vi "TestExec.File Sync Config.vi"(9 "Dialog":bool, 11 "Config Folder":path=path "C:/MTE/Test Executive/Config") -> (1 "Changed":bool)   [LabVIEW 2018]
uses:
  TestExec.File Sync Config Data.ctl
  <vilib>/KATE/Queues/Queue Utils.lvlib
  <vilib>/KATE/Files/File Utils.lvlib
panel:
  out "Tab Control":enum32{"Inputs", "Data", "Outputs"}(tab)=enum."Data"
  out "CfgFileExists":bool
  in  "Sync Now":bool
  in  "Sync Enabled":bool
  in  "Sync Items":T1(array[cluster])
  in  "Save":bool
  in  "Cancel":bool
  out "Sync Config File":path
  in  "Reload":bool
  out "Sync Config":T2
  # "File Sync Config"
  # "Path Types:\nSource    \tDestination     \tOutcome\nFILE          \tFILE\t\t                  The source file will be copied to the destination file.\nFILE\t     \t    FOLDER\t\t          The source file will be copied into the destination folder.\nFOLDER\t   FOLDER\t\t          All files and subfolders of the source folder will be copied into the destination folder. \nFOLDER\t   FILE\t            \t     This is an invalid combination.  An error will be generated."
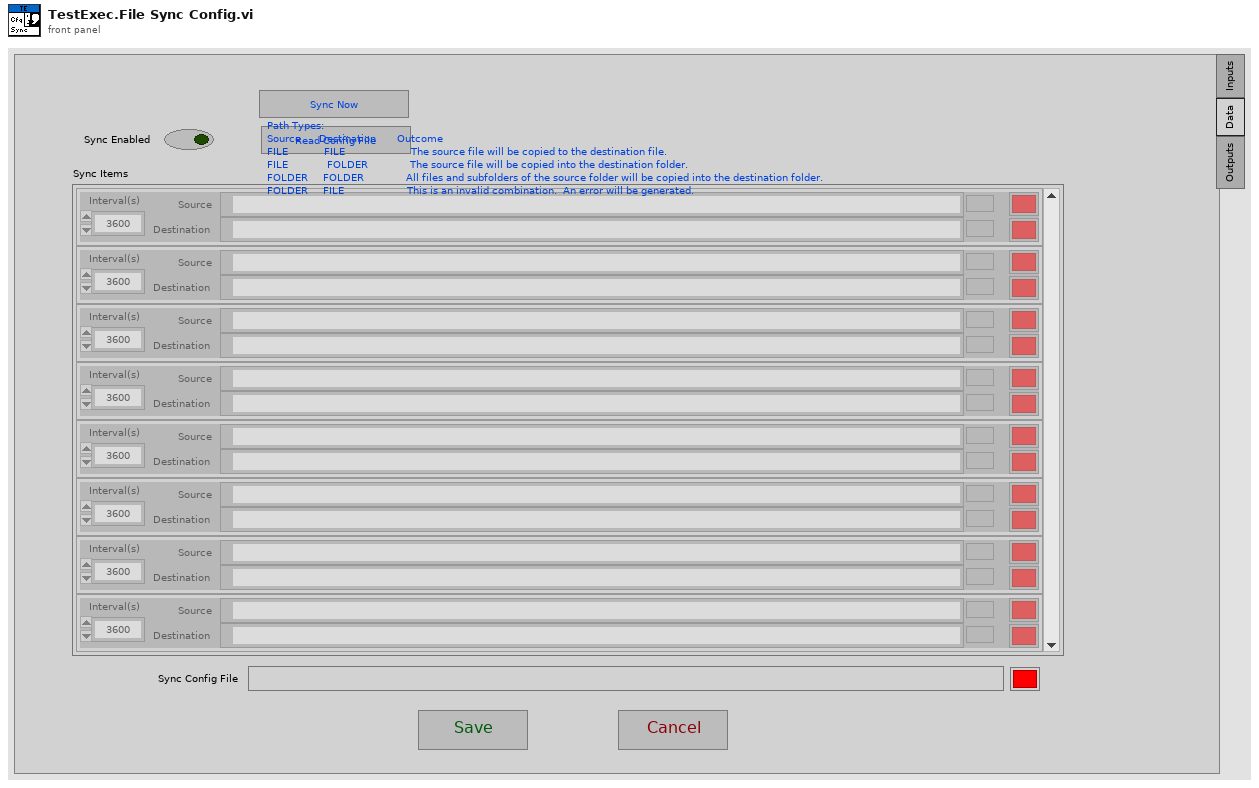
[diagram p1: front panel]
types:
  T1 = cluster{"Interval(s)":dbl, "Source":path, "Destination":path, "DestExists":bool, "SourceExists":bool}[]
  T2 = typedef "TestExec.File Sync Config Data.ctl" = cluster{"SyncEnabled":bool, "SyncItems":cluster{"Interval(s)":dbl, "Source":path, "Destination":path}[]}
  T3 = enum32{"Invalid", "Standard", "Closed", "Hidden", "Minimized", "Maximized"}
  T4 = cluster{"Enable":bool, "Files":cluster{"Interval":dbl, "Source":string, "Destination":string}[]}
  T5 = cluster{"Interval":dbl, "Source":string, "Destination":string}
  T6 = cluster{"Interval(s)":dbl, "Source":path, "Destination":path}
  T7 = cluster{"Interval(s)":dbl, "Source":path, "Destination":path, "DestExists":bool, "SourceExists":bool}
  T8 = cluster{"Config Folder":path, "Config File":path, "Sync Config":T2, "Canceled":bool}
  T9 = cluster{"Interval":dbl, "Source":string, "Destination":string}[]
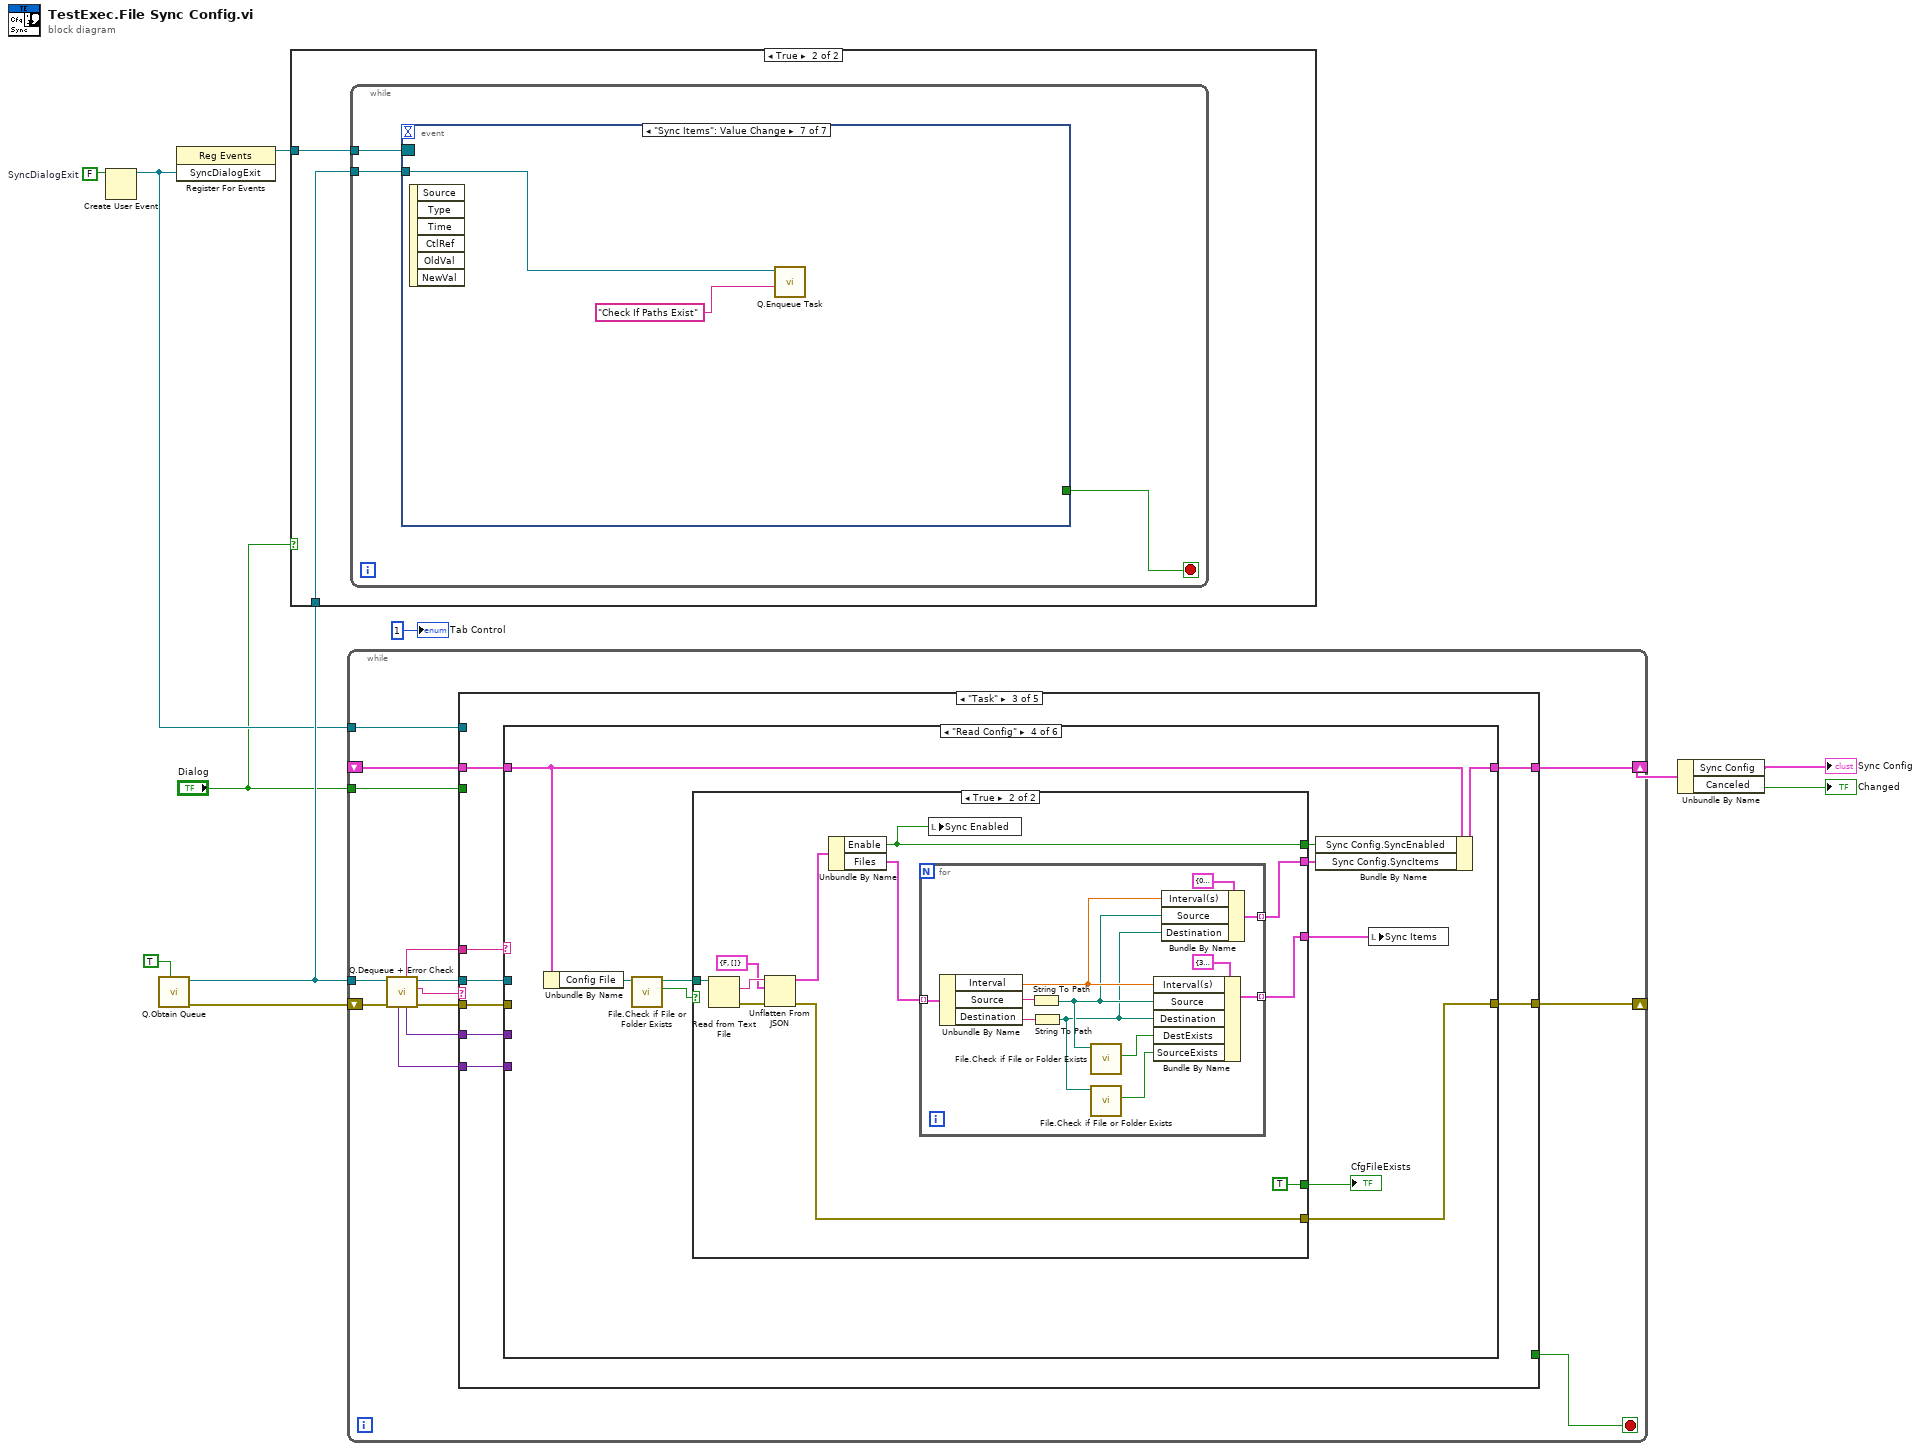
[diagram p0: block diagram]
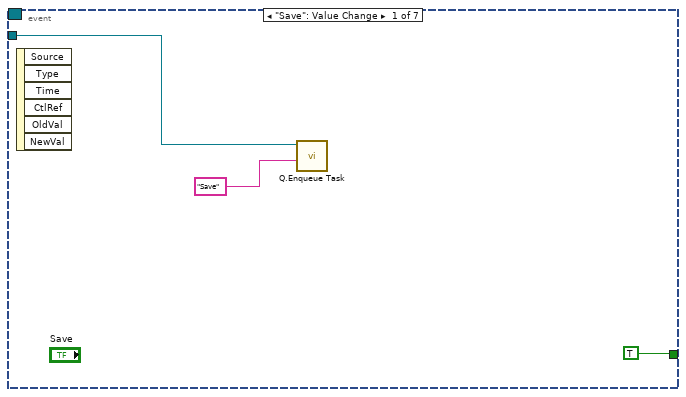
[diagram p3: hidden frame]
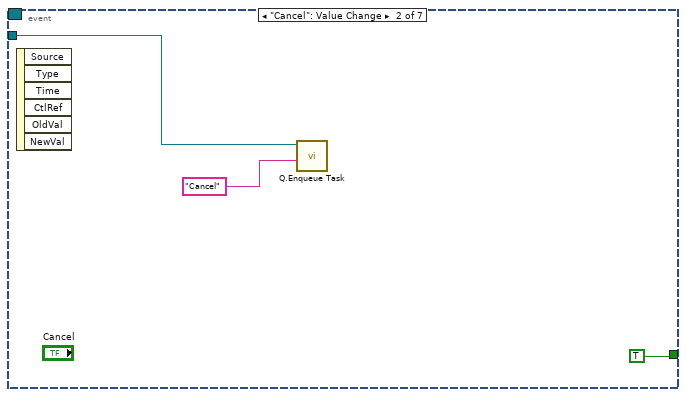
[diagram p4: hidden frame]
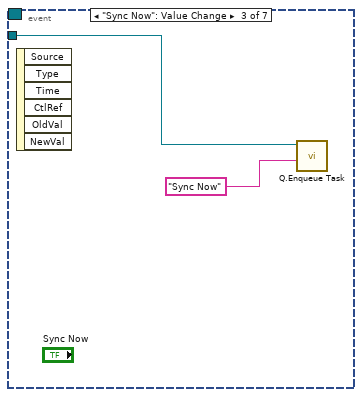
[diagram p5: hidden frame]
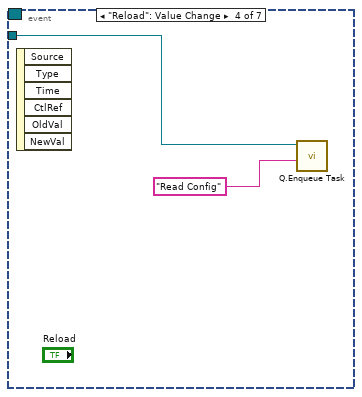
[diagram p6: hidden frame]
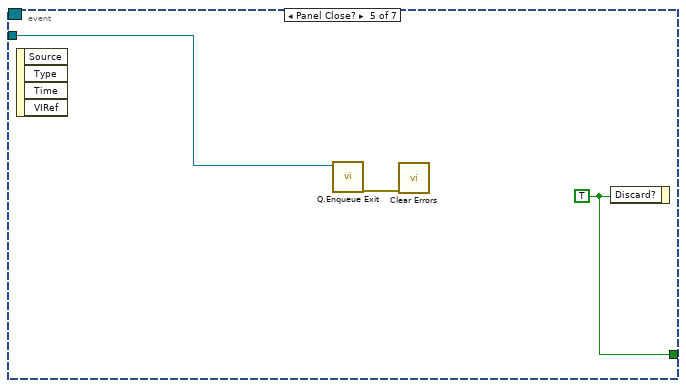
[diagram p7: hidden frame]
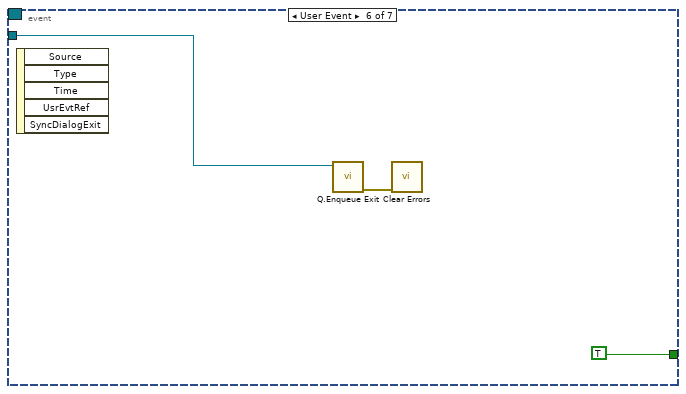
[diagram p8: hidden frame]
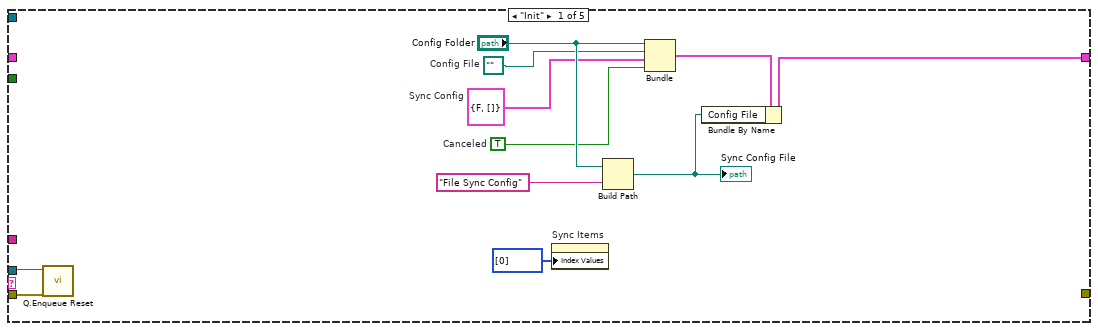
[diagram p9: hidden frame]
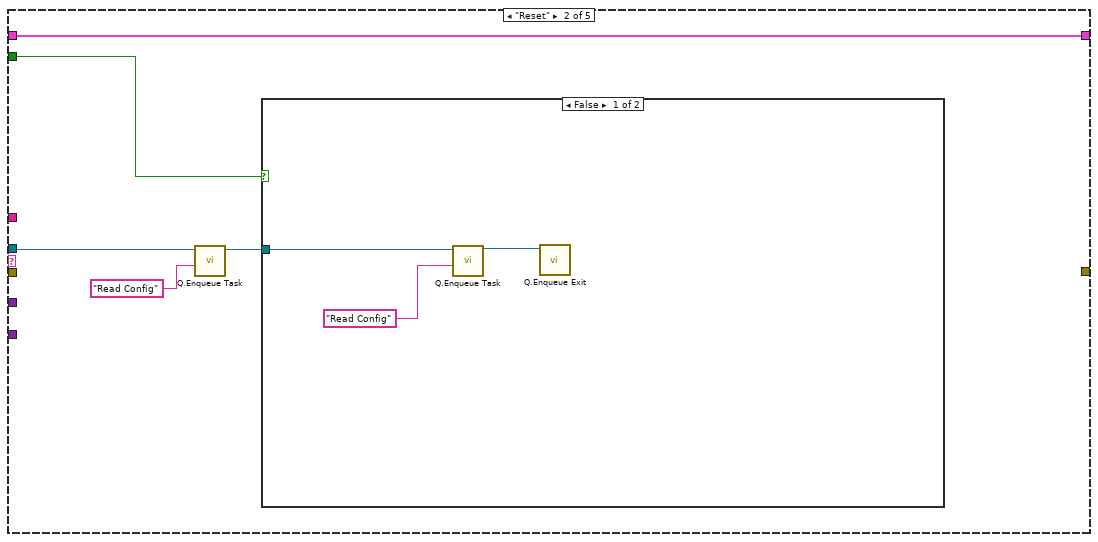
[diagram p10: hidden frame]
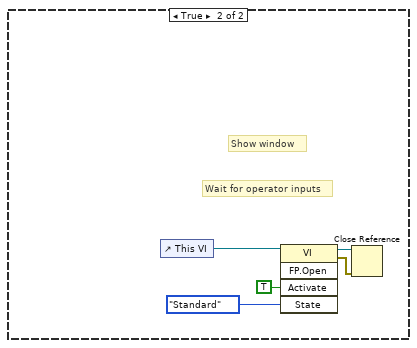
[diagram p11: hidden frame]
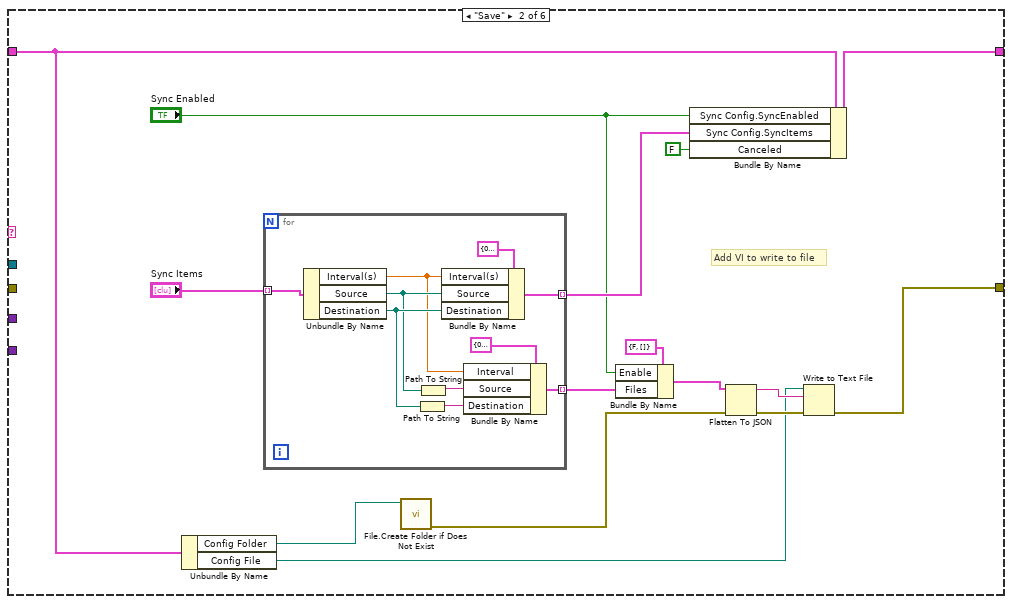
[diagram p13: hidden frame]
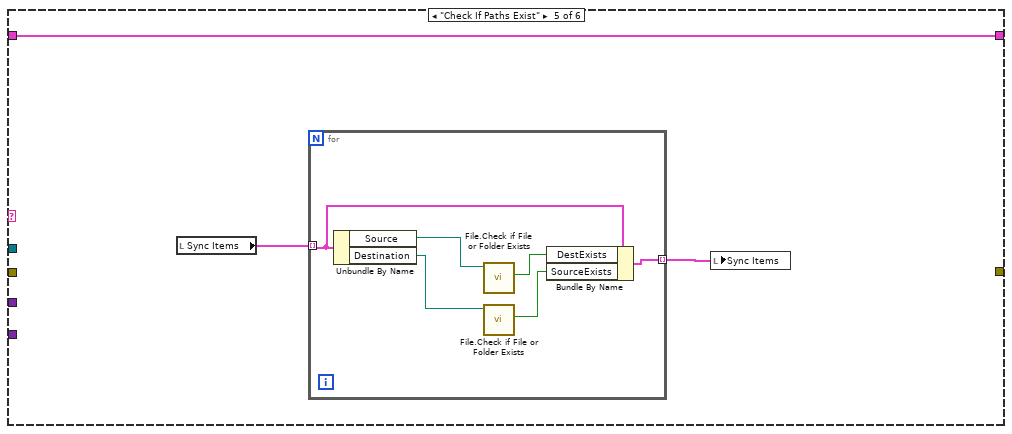
[diagram p16: hidden frame]
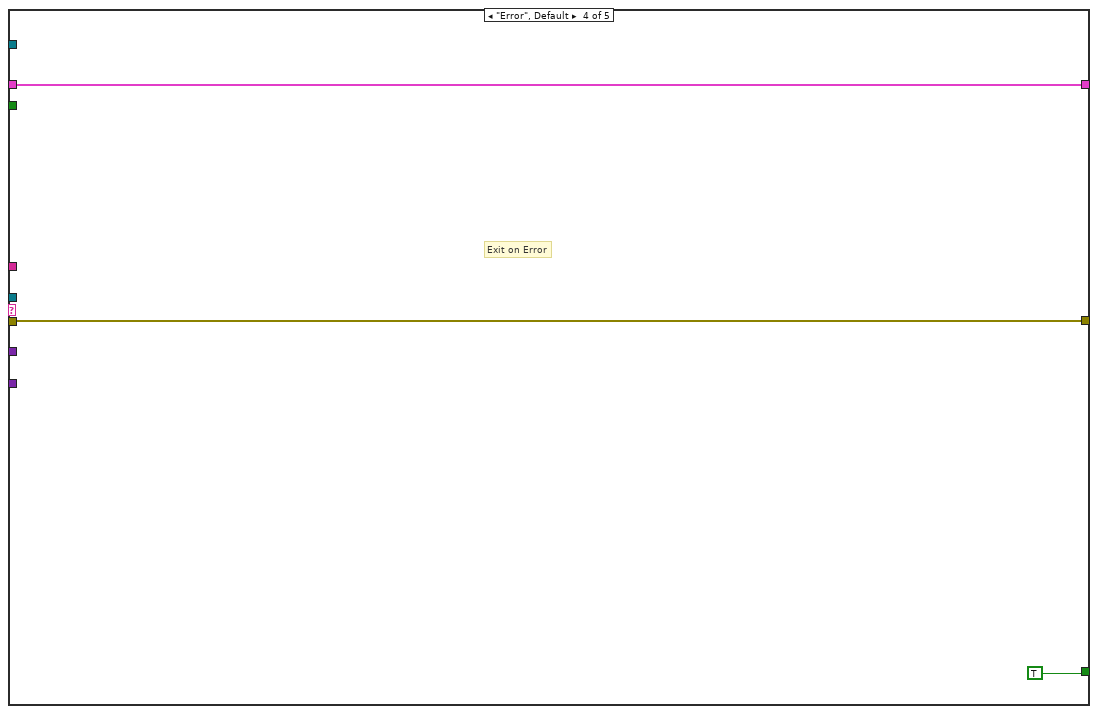
[diagram p18: hidden frame]
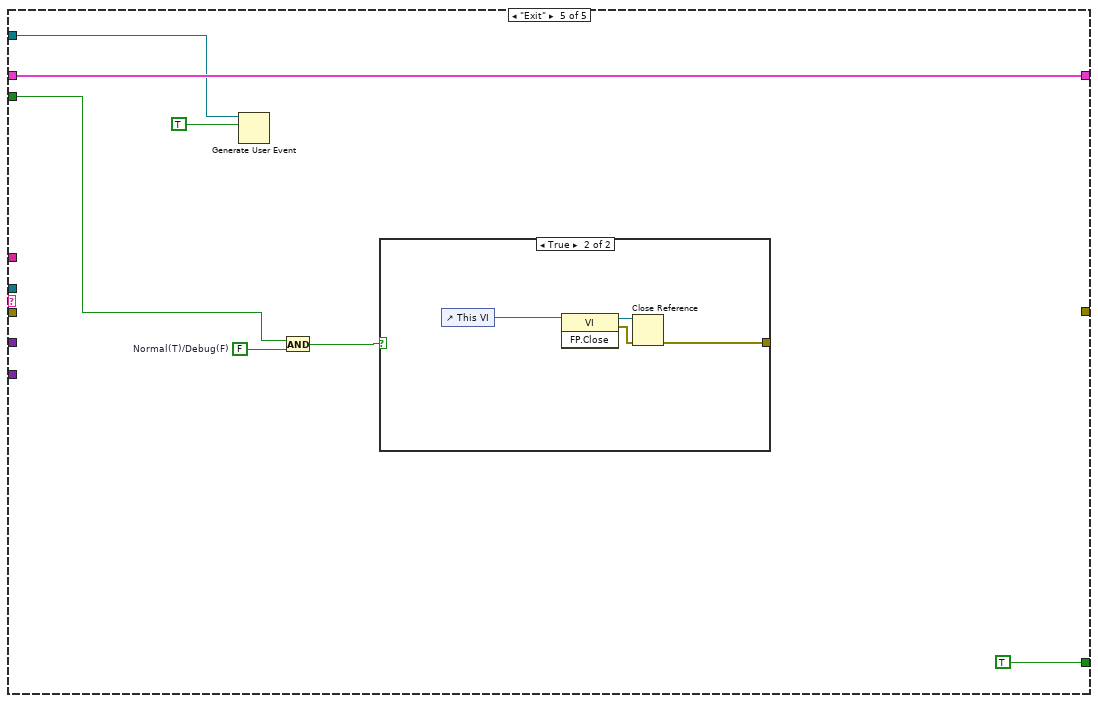
[diagram p19: hidden frame]
diagram:
  w11 = FALSE  # SyncDialogExit
  n1 = Create User Event(user event datatype=w11) -> (user event=w5:refnum<user-event>)  [unwired: 1 in, 1 out]
  n2 = call <vilib>:"Q.Obtain Queue.vi"("Enqueue Init"=TRUE) -> ("error out"=w7:errorcluster, "Q Out"=w6:refnum<queue>)  [unwired: 8 in, 1 out]
  n3 = register-events(w5) -> (reference out=w10:refnum<event-registration>)  [unwired: 2 in, 1 out]
  n4 = case shown="True" "Dialog" {
    tunnel: w10 -> [_ w13]
    tunnel: w6 -> [_ w12]
    frame False {
    }
    frame True {
      n5 = while {
        tunnel: w13 -> [w16]
        tunnel: w12 -> [w15]
        stop <- w14 stop-if-true
        n6 = event shown="[6] \"Sync Items\": Value Change" {
          selector: w16 -> [_ _ _ _ _ _ _]
          dyn-events: _ -> [_ _ _ _ _ _ _]
          timeout: _ -> [_ _ _ _ _ _ _]
          tunnel: w15 -> [w18 w21 w23 w25 w28 w31 w33]
          tunnel: [TRUE TRUE _ _ w29 TRUE _] -> w14
          event "Save": Value Change {
            n7 = event-data() -> ()  [unwired: 1 in, 6 out]
            n8 = call <vilib>:"Q.Enqueue Task.vi"("Task Name"="Save", "Q In"=w18) -> ()  [unwired: 8 in, 2 out]
          }
          event "Cancel": Value Change {
            n9 = event-data() -> ()  [unwired: 1 in, 6 out]
            n10 = call <vilib>:"Q.Enqueue Task.vi"("Task Name"="Cancel", "Q In"=w21) -> ()  [unwired: 8 in, 2 out]
          }
          event "Sync Now": Value Change {
            n11 = event-data() -> ()  [unwired: 1 in, 6 out]
            n12 = call <vilib>:"Q.Enqueue Task.vi"("Task Name"="Sync Now", "Q In"=w23) -> ()  [unwired: 8 in, 2 out]
          }
          event "Reload": Value Change {
            n13 = event-data() -> ()  [unwired: 1 in, 6 out]
            n14 = call <vilib>:"Q.Enqueue Task.vi"("Task Name"="Read Config", "Q In"=w25) -> ()  [unwired: 8 in, 2 out]
          }
          event Panel Close? {
            w29 = TRUE
            n15 = event-data() -> ()  [unwired: 1 in, 4 out]
            n16 = call <vilib>:"Q.Enqueue Exit.vi"("Q In"=w28) -> ("error out"=w27:errorcluster)  [unwired: 9 in, 1 out]
            n17 = call <vilib>:"Clear Errors.vi"("error in (no error)"=w27) -> ()  [unwired: 5 in, 2 out]
            n18 = event-data("Discard?"=w29) -> ()  [unwired: 1 in, 1 out]
          }
          event User Event {
            n19 = event-data() -> ()  [unwired: 1 in, 5 out]
            n20 = call <vilib>:"Q.Enqueue Exit.vi"("Q In"=w31) -> ("error out"=w30:errorcluster)  [unwired: 9 in, 1 out]
            n21 = call <vilib>:"Clear Errors.vi"("error in (no error)"=w30) -> ()  [unwired: 5 in, 2 out]
          }
          event "Sync Items": Value Change {
            n22 = event-data() -> ()  [unwired: 1 in, 6 out]
            n23 = call <vilib>:"Q.Enqueue Task.vi"("Task Name"="Check If Paths Exist", "Q In"=w33) -> ()  [unwired: 8 in, 2 out]
          }
        }
      }
    }
  }
  n24 = while {
    shift-right: [w40] -> _
    shift-left: w7 -> [w45]
    tunnel: w6 -> [w43]
    shift-right: [w38] -> w4
    shift-left: _ -> [w37]
    tunnel: w5 -> [w36]
    tunnel: "Dialog" -> [w35]
    stop <- w39 stop-if-true
    n25 = call <vilib>:"Q.Dequeue + Error Check.vi"("Error In"=w45, "Q In"=w43) -> ("error out"=w46:errorcluster, "Cmd"=w48:string, "Q Out"=w47:refnum<queue>, "Data1"=w42:variant, "Sub"=w44:string, "Data2"=w41:variant)  [unwired: 4 in]
    n26 = case shown="\"Task\"" w48 {
      tunnel: w47 -> [w49 w63 w79 _ _]
      tunnel: w46 -> [w50 _ w78 w152 _]
      tunnel: w44 -> [_ _ w80 _ _]
      tunnel: w42 -> [_ _ w77 _ _]
      tunnel: w41 -> [_ _ w76 _ _]
      tunnel: [_ _ w73 w152 _] -> w40
      tunnel: [_ _ _ TRUE TRUE] -> w39
      tunnel: [w58 w60 w74 w153 w159] -> w38
      tunnel: w37 -> [_ w60 w75 w153 w159]
      tunnel: w36 -> [_ _ _ _ w158]
      tunnel: w35 -> [_ w61 _ _ w154]
      frame "Init" {
        w52 = TRUE  # Canceled
        w55 = T2 {"SyncEnabled"=FALSE, "SyncItems"=[]}  # Sync Config
        w56 = path ""  # Config File
        n27 = call <vilib>:"Q.Enqueue Reset.vi"("Error In"=w50, "Q In"=w49) -> ()  [unwired: 8 in, 2 out]
        n28 = property on="Sync Items" class="Arr (strict)"("Index Values"=u32[] [0]) -> ()  [unwired: 2 in, 2 out]
        n29 = Build Path(base path="Config Folder", name or relative path="File Sync Config") -> (appended path=w54:path)
        "Sync Config File" <- w54
        n30 = Bundle("Config Folder"="Config Folder", "Config File"=w56, "Sync Config"=w55, "Canceled"=w52) -> (w59:T8)  [unwired: 1 in]
        n31 = Bundle By Name(cluster=w59, "Config File"=w54) -> (w58:T8)
      }
      frame "Reset" {
        n32 = call <vilib>:"Q.Enqueue Task.vi"("Task Name"="Read Config", "Q In"=w63) -> ("Q Out"=w62:refnum<queue>)  [unwired: 8 in, 1 out]
        n33 = case shown="False" w61 {
          tunnel: w62 -> [w66 _]
          frame False {
            n34 = call <vilib>:"Q.Enqueue Task.vi"("Task Name"="Read Config", "Q In"=w66) -> ("Q Out"=w65:refnum<queue>)  [unwired: 8 in, 1 out]
            n35 = call <vilib>:"Q.Enqueue Exit.vi"("Q In"=w65) -> ()  [unwired: 9 in, 2 out]
          }
          frame True {
            # "Show window"
            # "Wait for operator inputs"
            n36 = control-ref of="This VI"() -> (w72:refnum<vi>)
            n37 = invoke class="VI" method="FP.Open"(reference=w72, "Activate"=TRUE ("Activate?"), "State"=T3."Standard") -> (reference out=w71:refnum<vi>, error out=w70:errorcluster)  [unwired: 2 in, 3 out]
            n38 = Close Reference(reference=w71, error in (no error)=w70) -> ()  [unwired: 1 out]
          }
        }
      }
      frame "Task" {
        n39 = case shown="\"Read Config\"" w80 {
          tunnel: w79 -> [_ _ _ _ _ _]
          tunnel: w78 -> [_ _ _ _ _ _]
          tunnel: w77 -> [_ _ _ _ _ _]
          tunnel: w76 -> [_ _ _ _ _ _]
          tunnel: w75 -> [w81 w92 w107 w114 w143 w150]
          tunnel: [w81 w96 w107 w113 w143 w150] -> w74
          tunnel: [_ w86 _ w117 _ _] -> w73
          frame "Sync Now" {
            # "Add VI to perform Sync"
          }
          frame "Save" {
            # "Add VI to write to file"
            n40 = Unbundle By Name(w92) -> ("Config Folder"=w91:path, "Config File"=w87:path)
            n41 = for {
              tunnel: [w105] -> w93 mode=indexing
              tunnel: "Sync Items" -> [w104] mode=indexing
              tunnel: [w97] -> w84 mode=indexing
              n42 = Unbundle By Name(w104) -> ("Interval(s)"=w98:dbl, "Source"=w102:path, "Destination"=w103:path)
              n43 = Path To String(path=w103) -> (string=w100:string)
              n44 = Path To String(path=w102) -> (string=w101:string)
              n45 = Bundle By Name(cluster=T6 {"Interval(s)"=0.0, "Source"=path "", "Destination"=path ""} ("Sunc Config Item"), "Interval(s)"=w98, "Source"=w102, "Destination"=w103) -> (w105:T6)
              n46 = Bundle By Name(cluster=T5 {"Interval"=0.0, "Source"="", "Destination"=""} ("Sunc Config Item"), "Interval"=w98, "Source"=w101, "Destination"=w100) -> (w97:T5)
            }
            n47 = call <vilib>:"File.Create Folder if Does Not Exist.vi"("Path"=w91) -> ("error out"=w90:errorcluster)  [unwired: 8 in, 2 out]
            n48 = Bundle By Name(cluster=T4 {"Enable"=FALSE, "Files"=[]}, "Enable"="Sync Enabled", "Files"=w84) -> (w82:T4)
            n49 = Bundle By Name(cluster=w92, "Sync Config.SyncEnabled"="Sync Enabled", "Sync Config.SyncItems"=w93, "Canceled"=FALSE) -> (w96:T8)
            n50 = Flatten To JSON(anything=w82, error in (no error)=w90) -> (JSON string=w88:string, 11:w89:errorcluster)  [unwired: 1 in]
            n51 = Write to Text File(file (use dialog)=w87, text=w88, error in=w89) -> (error out=w86:errorcluster)  [unwired: 1 in, 2 out]
          }
          frame "Cancel" {
          }
          frame "Read Config" {
            n52 = Unbundle By Name(w114) -> ("Config File"=w111:path)
            n53 = call <vilib>:"File.Check if File or Folder Exists.vi"("Path"=w111) -> ("Exists"=w109:bool, "Dup Path"=w110:path)  [unwired: 6 in, 3 out]
            n54 = case shown="True" w109 {
              tunnel: [_ w123] -> w117
              tunnel: [_ w122] -> w116
              tunnel: [_ w121] -> w115
              tunnel: [_ w120] -> w112
              tunnel: w110 -> [_ w119]
              tunnel: [_ TRUE] -> w108
              frame False {
              }
              frame True {
                n55 = Read from Text File(file (use dialog)=w119) -> (text=w128:string, error out=w126:errorcluster)  [unwired: 3 in, 2 out]
                n56 = Unflatten From JSON(JSON string=w128, type and defaults=T4 {"Enable"=FALSE, "Files"=[]}, error in (no error)=w126) -> (value=w125:T4, error out=w123:errorcluster)  [unwired: 4 in]
                n57 = Unbundle By Name(w125) -> ("Enable"=w121:bool, "Files"=w124:T9)
                n58 = for {
                  tunnel: w124 -> [w140] mode=indexing
                  tunnel: [w136] -> w122 mode=indexing
                  tunnel: [w132] -> w120 mode=indexing
                  n59 = Unbundle By Name(w140) -> ("Interval"=w131:dbl, "Source"=w138:string, "Destination"=w137:string)
                  n60 = String To Path(string=w138) -> (path=w130:path)
                  n61 = String To Path(string=w137) -> (path=w129:path)
                  n62 = call <vilib>:"File.Check if File or Folder Exists.vi"("Path"=w130) -> ("Exists"=w135:bool)  [unwired: 6 in, 4 out]
                  n63 = call <vilib>:"File.Check if File or Folder Exists.vi"("Path"=w129) -> ("Exists"=w134:bool)  [unwired: 6 in, 4 out]
                  n64 = Bundle By Name(cluster=T7 {"Interval(s)"=3600.0, "Source"=path "", "Destination"=path "", "DestExists"=FALSE, "SourceExists"=FALSE} ("Sunc Config Item"), "Interval(s)"=w131, "Source"=w130, "Destination"=w129, "DestExists"=w135, "SourceExists"=w134) -> (w136:T7)
                  n65 = Bundle By Name(cluster=T6 {"Interval(s)"=0.0, "Source"=path "", "Destination"=path ""} ("Sunc Config Item"), "Interval(s)"=w131, "Source"=w130, "Destination"=w129) -> (w132:T6)
                }
                n66 = local write "Sync Enabled"(w121) -> ()
              }
            }
            "CfgFileExists" <- w108
            n67 = Bundle By Name(cluster=w114, "Sync Config.SyncEnabled"=w115, "Sync Config.SyncItems"=w112) -> (w113:T8)
            n68 = local write "Sync Items"(w116) -> ()
          }
          frame "Check If Paths Exist" {
            n69 = local read "Sync Items"() -> (w142:T1)
            n70 = for {
              tunnel: w142 -> [w144] mode=indexing
              tunnel: [w145] -> w141 mode=indexing
              n71 = Unbundle By Name(w144) -> ("Source"=w147:path, "Destination"=w146:path)
              n72 = call <vilib>:"File.Check if File or Folder Exists.vi"("Path"=w147) -> ("Exists"=w149:bool)  [unwired: 6 in, 4 out]
              n73 = call <vilib>:"File.Check if File or Folder Exists.vi"("Path"=w146) -> ("Exists"=w148:bool)  [unwired: 6 in, 4 out]
              n74 = Bundle By Name(cluster=w144, "DestExists"=w149, "SourceExists"=w148) -> (w145:T7)
            }
            n75 = local write "Sync Items"(w141) -> ()
          }
          frame Default {
          }
        }
      }
      frame "Error", Default {
        # "Exit on Error"
      }
      frame "Exit" {
        w155 = FALSE  # Normal(T)/Debug(F)
        n76 = Generate User Event(user event=w158, event data cluster=TRUE ("event data")) -> ()  [unwired: 2 in, 2 out]
        n77 = And(x=w154, y=w155) -> (x .and. y?=w156:bool)
        n78 = case shown="True" w156 {
          tunnel: [_ w161] -> _
          frame False {
          }
          frame True {
            n79 = control-ref of="This VI"() -> (w164:refnum<vi>)
            n80 = invoke class="VI" method="FP.Close"(reference=w164) -> (reference out=w163:refnum<vi>, error out=w162:errorcluster)  [unwired: 2 in, 1 out]
            n81 = Close Reference(reference=w163, error in (no error)=w162) -> (error out=w161:errorcluster)
          }
        }
      }
    }
  }
  n82 = Unbundle By Name(w4) -> ("Sync Config"=→"Sync Config":T2, "Canceled"=→"Changed":bool)
  "Tab Control" <- 1
